vi "ITX to LV 2.1.vi"(0 "file (use dialog)":path=path "P:/sample/GaAs/GaAs quantum dots/2008/PL Map/A1 735/060731ASBA_A1_6.0.itx") -> (2 "2D array":dbl[][](array[numeric]), 3 "1D arrays":dbl[][](array[numeric]), 4 "wave names":string[](array[string]), 5 "Notes":string)   [LabVIEW 2011]
panel:
  out "1D array":dbl[][](graph)
  out "2D array":dbl[][](graph)
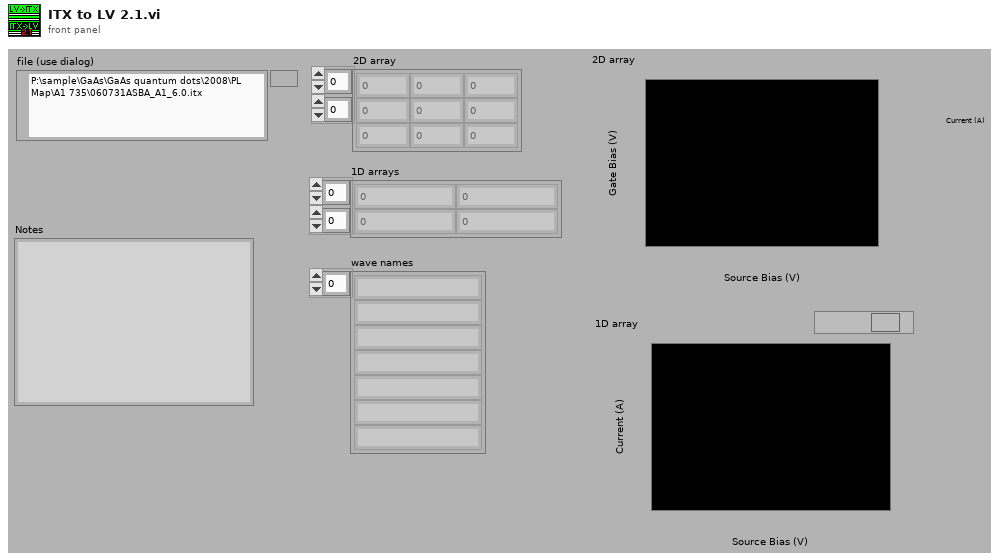
[diagram p1: front panel]
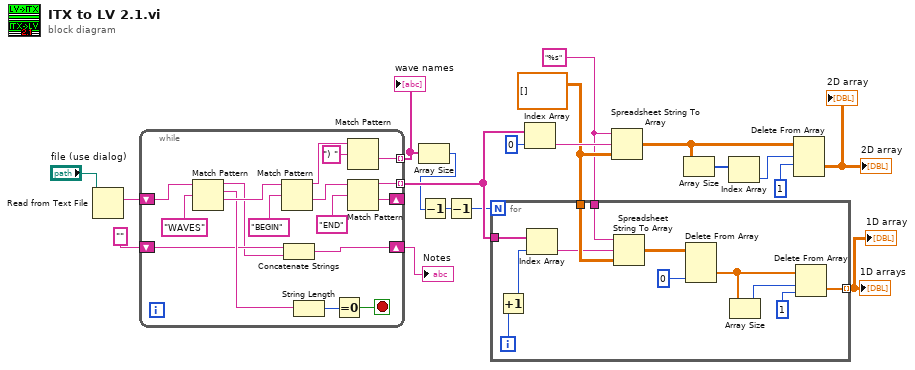
[diagram p0: block diagram]
diagram:
  w8 = "%s" ("format string")
  w11 = dbl[][] [] ("array type (2D Dbl)")
  n1 = Read from Text File(file (use dialog)="file (use dialog)") -> (text=w19:string)  [unwired: 2 in, 4 out]
  n2 = while {
    tunnel: [w33] -> w10 mode=indexing
    shift-right: [w34] -> _
    shift-left: w19 -> [w21]
    tunnel: [w29] -> w5 mode=indexing
    shift-right: [w24] -> w9
    shift-left: "" ("regular expression") -> [w23]
    stop <- w30 stop-if-true
    n3 = Match Pattern(string=w21, regular expression="WAVES") -> (before substring=w22:string, match substring=w32:string, after substring=w36:string)  [unwired: 2 out]
    n4 = Match Pattern(string=w36, regular expression="BEGIN" ("regular expression 2")) -> (before substring=w20:string, after substring=w35:string)  [unwired: 3 out]
    n5 = Concatenate Strings(w23, w22) -> (w24:string)
    n6 = String Length(string=w32) -> (length=w31:i32)
    n7 = Equal To 0?(x=w31) -> (x = 0?=w30:bool)
    n8 = Match Pattern(string=w20, regular expression=") ") -> (after substring=w29:string)  [unwired: 4 out]
    n9 = Match Pattern(string=w35, regular expression="END" ("regular expression 3")) -> (before substring=w33:string, after substring=w34:string)  [unwired: 3 out]
  }
  "wave names" <- w5
  "Notes" <- w9
  n10 = Array Size(array=w5) -> (size(s)=w4:i32)
  n11 = Decrement(x=w4) -> (x-1=w7:i32)
  n12 = Decrement(x=w7) -> (x-1=w6:i32)
  n13 = for {
    N: w6 -> [_]
    tunnel: [w46] -> w1 mode=indexing
    tunnel: w11 -> [w42]
    tunnel: w10 -> [w41]
    tunnel: w8 -> [w40]
    i -> [w39]
    n14 = Increment(x=w39) -> (x+1=w38:i32)
    n15 = Index Array(array=w41, index=w38) -> (element=w37:string)
    n16 = Spreadsheet String To Array(format string=w40, spreadsheet string=w37, array type (2D Dbl)=w42) -> (array=w47:dbl[][])  [unwired: 1 out]
    n17 = Delete From Array(array=w47, index (col)=0 ("disabled index (col)")) -> (deleted portion=w45:dbl[])  [unwired: 2 in, 1 out]
    n18 = Array Size(array=w45) -> (size(s)=w44:i32)
    n19 = Delete From Array(array=w45, length=w44, index=1) -> (deleted portion=w46:dbl[])  [unwired: 1 out]
  }
  "1D arrays" <- w1
  "1D array" <- w1
  n20 = Index Array(array=w10, index=0) -> (element=w17:string)
  n21 = Spreadsheet String To Array(format string=w8, spreadsheet string=w17, array type (2D Dbl)=w11) -> (array=w15:dbl[][])  [unwired: 1 out]
  n22 = Array Size(array=w15) -> (size(s)=w14:i32[])
  n23 = Index Array(array=w14) -> (element=w12:i32)  [unwired: 1 in]
  n24 = Delete From Array(array=w15, length=w12, index (row)=1) -> (deleted portion=→"2D array" →"2D array":dbl[][])  [unwired: 1 in, 1 out]
